vi "Parameters Import Action - Create Chans.vi"(8 "error in (no error)":errorcluster, 10 "selected path":path, 11 "Node Ptr":u64) -> (0 "error out":errorcluster, 2 "selected path out":path caption="selected path", 3 "Node Ptr dup":u64)   [LabVIEW 2019, in "Ballard Arinc-429 System Explorer.lvlib"]
uses:
  Ballard Arinc-429 System Explorer.lvlib
  Create Sysdef Tree from Parameters Clusters_Find Label Refs.vi
  Create Sysdef Tree from Parameters Clusters_Find Channel Ref.vi
  Shared/Controls and Global/Global.vi
  <vilib>/NI VeriStand/Custom Device Tools/Custom Device Utility Library/NI VeriStand - Search for Item.vi
  <vilib>/NI VeriStand/Custom Device Tools/Custom Device Utility Library/NI VeriStand - Search for Item by GUID.vi
  <vilib>/NI VeriStand/Custom Device Tools/Custom Device Utility Library/NI VeriStand - Search for All Items by GUID.vi
  <vilib>/NI VeriStand/Custom Device API/NI VeriStand - Get Item Property.vi
  <vilib>/NI VeriStand/Custom Device API/Get Item Property (U16).vi
  <vilib>/NI VeriStand/Custom Device API/NI VeriStand - Get Item Children.vi
  <vilib>/NI VeriStand/Custom Device API/Get Item Property (U32).vi
  <vilib>/NI VeriStand/Custom Device API/Get Item Property (Boolean).vi
  <vilib>/NI VeriStand/Custom Device API/NI VeriStand - Get Item Data.vi
  <vilib>/NI VeriStand/Custom Device Tools/Custom Device Utility Library/NI VeriStand - Get All Channels.vi
  <vilib>/NI VeriStand/Custom Device API/NI VeriStand - Remove Custom Device Item.vi
  AddParamChannels.vi
  <vilib>/NI VeriStand/Custom Device API/Custom Device API.lvlib
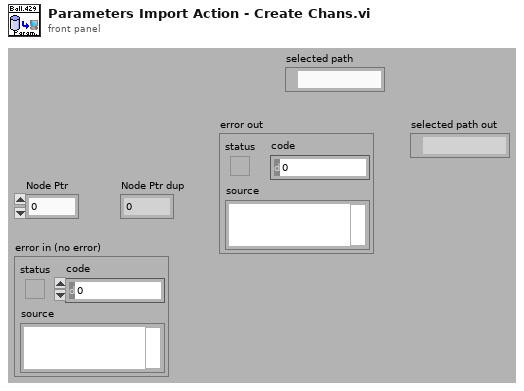
[diagram p1: front panel]
types:
  T1 = typedef "XML_Channel.ctl" = cluster{"hardwareChannel":i32, "Labels":T2[]}
  T2 = typedef "XML_Label.ctl" = cluster{"labelDecimal":i32, "Parameters":T3[], "createSDIChannel":bool, "createSSMChannel":bool, "createParityChannel":bool, "SDI_Enabled":bool, "SDIValue":u8}
  T3 = typedef "XML_Parameter.ctl" = cluster{"encoding":enum16{"BNR", "BCD", "Discrete"}, "signed":bool, "startBit":i32, "numberOfBits":i32, "scale":dbl, "offset":dbl, "names":string[], "defaultValues":dbl[], "Unit":string}
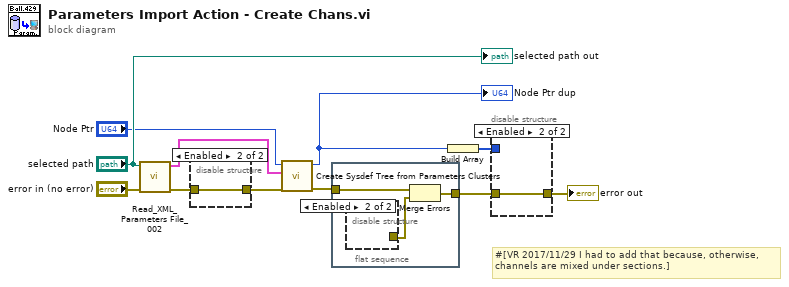
[diagram p0: block diagram]
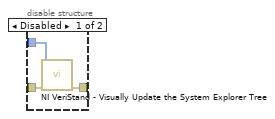
[diagram p2: hidden frame]
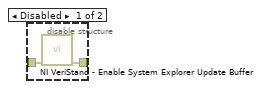
[diagram p3: hidden frame]
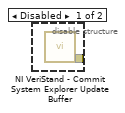
[diagram p4: hidden frame]
diagram:
  # "#[VR 2017/11/29 I had to add that because, otherwise,\nchannels are mixed under sections.]"
  n1 = call "Read_XML_Parameters File_002.vi"("error in (no error)"="error in (no error)", "XML Configuration File Path"="selected path") -> ("error out"=w9:errorcluster, "Channels"=w5:T1[])  [unwired: 8 in]
  n2 = disable-structure shown="Enabled" {
    disable-tunnel: w9 -> [w13 w14]
    disable-tunnel: [w12 w14] -> w4
    frame Disabled {
      n3 = call <vilib>:"NI VeriStand - Enable System Explorer Update Buffer.vi"("error in (no error)"=w13) -> ("error out"=w12:errorcluster)  [unwired: 10 in]
    }
    frame Enabled {
    }
  }
  n4 = call "Create Sysdef Tree from Parameters Clusters.vi"("error in"=w4, "Channels"=w5, "Device Ptr"="Node Ptr") -> ("error out"=w1:errorcluster, "Device Ptr dup"=w2:u64)  [unwired: 7 in]
  "Node Ptr dup" <- w2
  n5 = flat-sequence {
    tunnel: w1 -> [w17]
    tunnel: [w15] -> w8
    frame #0 {
      n6 = disable-structure shown="Enabled" {
        disable-tunnel: [w18 _] -> w16
        frame Disabled {
          n7 = call <vilib>:"NI VeriStand - Commit System Explorer Update Buffer.vi"() -> ("error out"=w18:errorcluster)  [unwired: 11 in]
        }
        frame Enabled {
        }
      }
      n8 = Merge Errors(w17, w16) -> (w15:errorcluster)
    }
  }
  n9 = Build Array(w2) -> (w6:u64[])
  n10 = disable-structure shown="Enabled" {
    disable-tunnel: w8 -> [w21 w22]
    disable-tunnel: [w20 w22] -> w7
    disable-tunnel: w6 -> [w19 _]
    frame Disabled {
      n11 = call "NI VeriStand - Visually Update the System Explorer Tree.vi"("error in (no error)"=w21, "Node IDs"=w19) -> ("error out"=w20:errorcluster)  [unwired: 9 in]
    }
    frame Enabled {
    }
  }
  "error out" <- w7
  "selected path out" <- "selected path"
